vi "niRFUtil CONV 1 Ohm Watt to dBm (complex array).vi"(7 "Complex Array (W)":T2 format="%.2f") -> (8 "Real Array (dBm)":T1 min=0 max=127 format="%.2f")   [LabVIEW 2015, in "niRFUtil.lvlib"]
doc: "(c) Copyright 2006, National Instruments, Inc. This VI may not be duplicated, sold, or distributed without written consent from National Instruments."
uses:
  niRFUtil.lvlib
  Includes/niRFUtil INC Complex Array.ctl
  Includes/niRFUtil INC Real Array.ctl
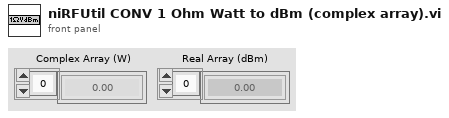
[diagram p1: front panel]
types:
  T1 = typedef "niRFUtil.lvlib/niRFUtil INC Real Array.ctl" = sgl[]
  T2 = typedef "niRFUtil.lvlib/niRFUtil INC Complex Array.ctl" = csg[]
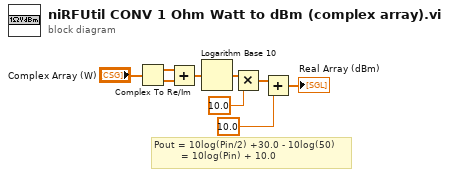
[diagram p0: block diagram]
diagram:
  # "Pout = 10log(Pin/2) +30.0 - 10log(50)\n         = 10log(Pin) + 10.0"
  n1 = Complex To Re/Im(x + iy="Complex Array (W)") -> (x=w5:sgl[], y=w4:sgl[])
  n2 = Add(x=w5, y=w4) -> (x+y=w3:sgl[])
  n3 = Logarithm Base 10(1:w3) -> (0:w9:sgl[])
  n4 = Multiply(x=w9, y=sgl 10.0) -> (x*y=w7:sgl[])
  n5 = Add(x=w7, y=sgl 10.0) -> (x+y=→"Real Array (dBm)":sgl[])
